vi "Resubmit Folder for static DOS.vi"() -> ()   [LabVIEW 2010]
panel:
  in  "Append":string="_DOS"
  in  "New DIrectory":path
  in  "Original Directory":path
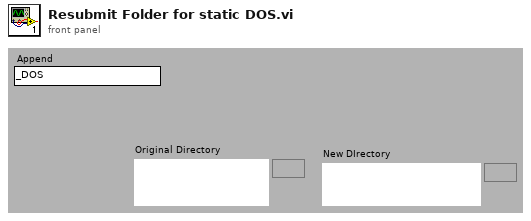
[diagram p1: front panel]
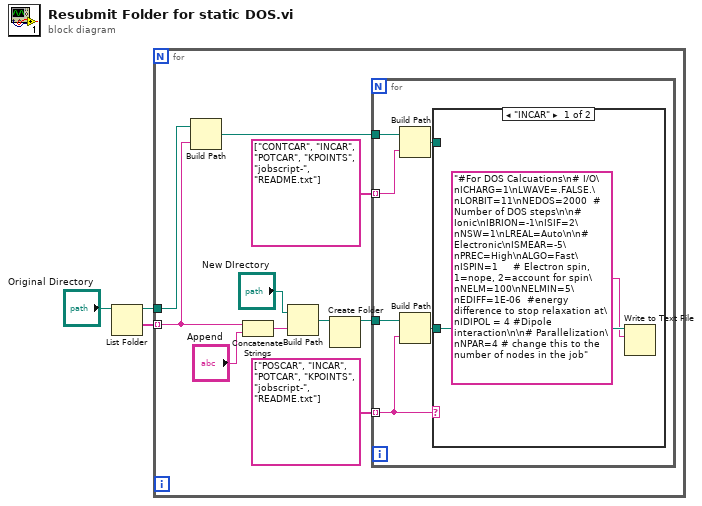
[diagram p0: block diagram]
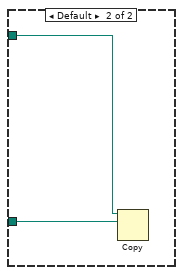
[diagram p2: hidden frame]
diagram:
  n1 = List Folder(path="Original Directory") -> (path out=w1:path, folder names=w2:string[])  [unwired: 3 in, 2 out]
  n2 = for {
    tunnel: w2 -> [w6] mode=indexing
    tunnel: w1 -> [w13]
    n3 = Build Path(base path=w13, name or relative path=w6) -> (appended path=w10:path)
    n4 = Concatenate Strings(w6, "Append") -> (w4:string)
    n5 = Build Path(base path="New DIrectory", name or relative path=w4) -> (appended path=w11:path)
    n6 = Create Folder(path (use dialog)=w11) -> (created path=w9:path)  [unwired: 2 in, 2 out]
    n7 = for {
      tunnel: w10 -> [w19]
      tunnel: w9 -> [w16]
      tunnel: string[] ["CONTCAR", "INCAR", "POTCAR", "KPOINTS", "jobscript-", "README.txt"] -> [w18] mode=indexing
      tunnel: string[] ["POSCAR", "INCAR", "POTCAR", "KPOINTS", "jobscript-", "README.txt"] -> [w14] mode=indexing
      n8 = Build Path(base path=w19, name or relative path=w18) -> (appended path=w17:path)
      n9 = Build Path(base path=w16, name or relative path=w14) -> (appended path=w15:path)
      n10 = case shown="\"INCAR\"" w14 {
        tunnel: w17 -> [_ w23]
        tunnel: w15 -> [w21 w22]
        frame "INCAR" {
          n11 = Write to Text File(file (use dialog)=w21, text="#For DOS Calcuations\n# I/O\nICHARG=1\nLWAVE=.FALSE.\nLORBIT=11\nNEDOS=2000  # Number of DOS steps\n\n# Ionic\nIBRION=-1\nISIF=2\nNSW=1\nLREAL=Auto\n\n# Electronic\nISMEAR=-5\nPREC=High\nALGO=Fast\nISPIN=1     # Electron spin, 1=nope, 2=account for spin\nNELM=100\nNELMIN=5\nEDIFF=1E-06  #energy difference to stop relaxation at\nIDIPOL = 4 #Dipole interaction\n\n# Parallelization\nNPAR=4 # change this to the number of nodes in the job") -> ()  [unwired: 2 in, 3 out]
        }
        frame Default {
          n12 = Copy(10:w22, 11:w23) -> ()  [unwired: 3 in, 3 out]
        }
      }
    }
  }
